vi "DIALOG_Cluster Item Selection.vi"(7 "Action":T4=enum."Bundler Insert", 8 "Error In":errorcluster, 9 "User VI Ref":refnum<vi>, 10 "Affected Items":T2, 11 "Display Items":T3[](array[typedef])) -> (0 "Error Out":errorcluster, 1 "Hide Full Names Out":bool=TRUE, 2 "Action Choice Out":enum32{"Choice 1", "Choice 2"}(radio), 3 "Selected Items (tags)":string[](array[string]))   [LabVIEW 2023]
doc: "Dialog to select items from the input cluster ref. \n\nFilter narrows list of items.\nDown key puts focus on tree and selects first item.\nUp and Down keps navigate tree.\nMultiple items can be selected.\n\nIn case of action \"Delete\" (\"Remove elements(s)...\" selected), list will show all elements currently displayed, else it will show all elements availabel to undle or unbundle.\n\nOutput is a list of the selected item tags.\n\nSelected element is the item clicked in a bundler node, displayed ot help user remember where an insert will happen."
uses:
  controls/Done Button.ctl
  controls/action enum.ctl
  cluster/Cluster Element Description.ctl
  top/BundleMagic.ctl
  utils/Controls/Get-Set Enum.ctl
  LabVIEW-common/String/Select All/String Select All CTRL-A_all string.vi
  <userlib>/_OpenG.lib/appcontrol/appcontrol.llb/openg_application_control.lvlib
  <userlib>/_OpenG.lib/error/error.llb/openg_error.lvlib
panel:
  in  "Filter":string
  in  "Tree":string[](tree)
  in  "Hide Full Names":bool=TRUE
  in  "Select Unwired":bool
  out "Selected Element String":string
  in  "Action Choice Radio Buttons":enum32{"Choice 1", "Choice 2"}(radio)
  in  "Done":T1
  in  "Show radio":bool
  in  "C1":T5
  # "All panes scroll to origin at runtime, so we don't have to worry about pane placements\n\nThis pane contracts at runtime and vertical splitter to left sticks to right at runtime so resizing functions happen as expected."
  # "Debug"
  # "Debug Cluster"
  # "(Use for debug if display items empty)"
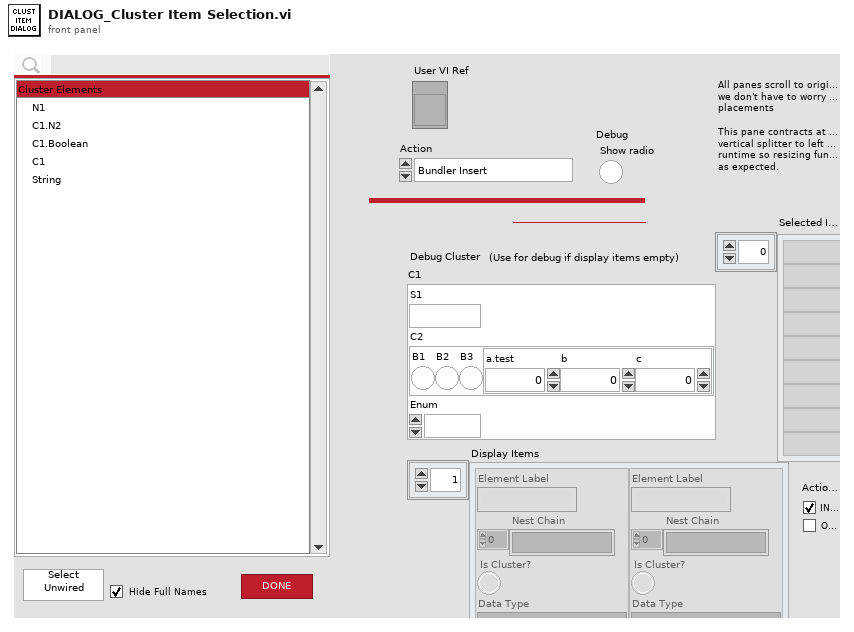
[diagram p1: front panel]
types:
  T1 = typedef "Done Button.ctl" = bool
  T2 = typedef "BundleMagic.ctl" = cluster{"Terminals":refnum<vi>[], "Wires":refnum<vi>[], "Named Bundler":refnum<vi>[], "Named Unbundler":refnum<vi>[], "In Place Cluster Node":refnum<vi>[], "Class Specifier Constant":refnum<vi>[], "Property Node":refnum<vi>[], "Invoke Node":refnum<vi>[], "Refnum Control":refnum<vi>[]}
  T3 = typedef "Cluster Element Description.ctl" = cluster{"Element Label":string, "Nest Chain":string[], "Is Cluster?":bool, "Data Type":variant, "Bundler Label":string, "Disabled":bool, "Unwired":bool, "Tree Tag":string}
  T4 = typedef "action enum.ctl" = enum16{"[NONE]", "APP_SEPARATOR", "Wire Bundle", "Wire Unbundle", "Terminal Unbundle", "Terminal Bundle", "Bundler Move Up", "Bundler Move Down", "Bundler Insert", "Bundler Remove", "Bundler Remove Unwired", "Bundler Reorder", "In Place Insert", "In Place Remove", "In Place Remove Unwired", "In Place Reorder", "Wire Properties", "Wire Method", "Terminal Properties", "Terminal Method", "Property Move Up", "Property Move Down", "Properties Insert", "Properties Remove", "Properties Remove Unwired", "Properties Reorder", "Method Change", "Class For Constant", "Class For Control", "Class For Node", "Class Name to Clipboard"}
  T5 = cluster{"S1":string, "C2":cluster{"B1":bool, "B2":bool, "B3":bool, cluster{"a.test":dbl, "b":i32, "c":u8}}, "Enum":enum16{""}}
  T6 = typedef "Get-Set Enum.ctl" = enum16{"Get", "Set"}
  T7 = typedef "LVPoint32TypeDef.ctl" = cluster{"Horizontal":i32, "Vertical":i32}
  T8 = cluster{"Shift":bool, "Ctrl":bool, "Alt":bool, "Cmd":bool, "Opt":bool}
  T9 = typedef "eventvkey.ctl" = enum16{"ASCII", "Enter", "Return", "Shift", "Ctrl", "Alt", "Cmd", "Opt", "Caps", "NumLock", "Clear", "Break", "Up", "Down", "Left", "Right", "Insert", "Delete", "Home", "End", "PageUp", "PageDown", "Escape", "Help", "Pause", "ScrollLock", "F1", "F2", "F3", "F4", "F5", "F6", "F7", "F8", "F9", "F10", "F11", "F12", "F13", "F14", "F15", "F16", "F17", "F18", "F19", "F20", "F21", "F22", "F23", "F24", "Play", "VolumeUp", "VolumeDown", "Mute", "Two Byte Char"}
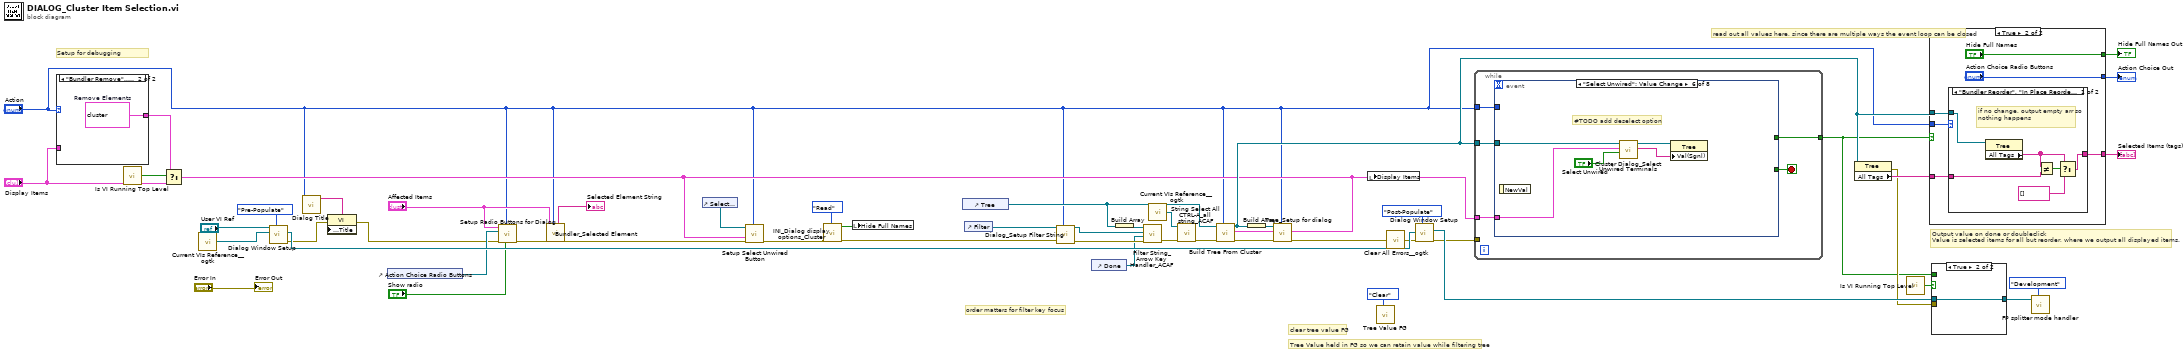
[diagram p0: block diagram]
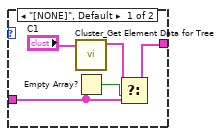
[diagram p2: hidden frame]
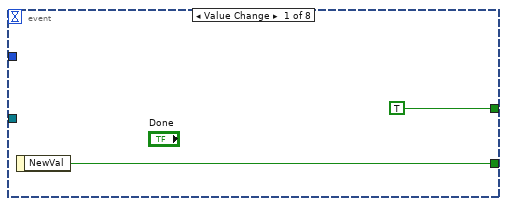
[diagram p3: hidden frame]
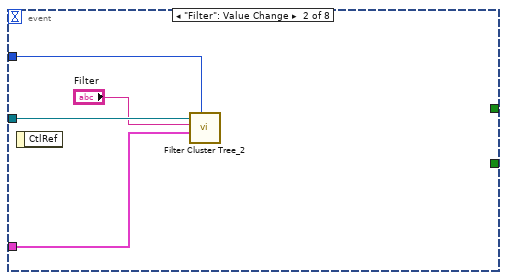
[diagram p4: hidden frame]
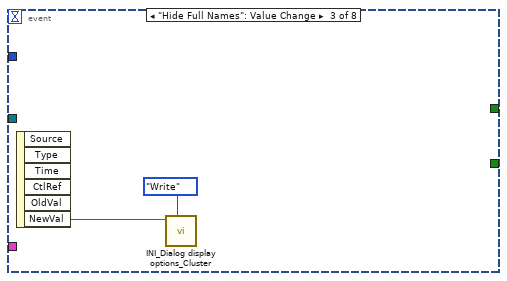
[diagram p5: hidden frame]
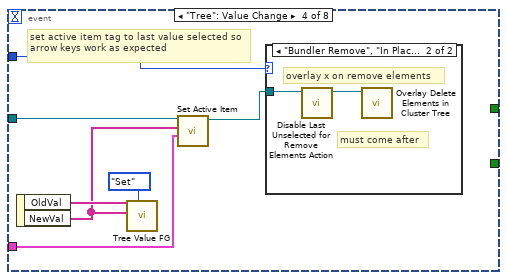
[diagram p6: hidden frame]
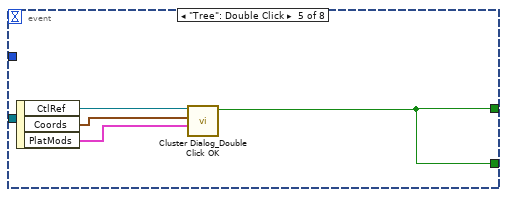
[diagram p8: hidden frame]
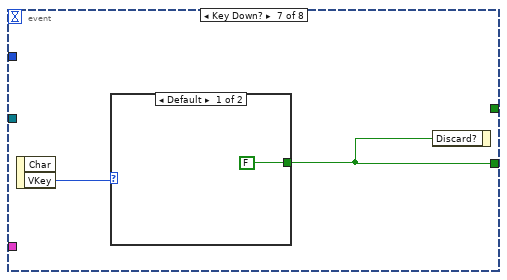
[diagram p9: hidden frame]
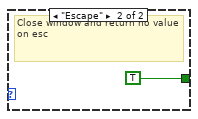
[diagram p10: hidden frame]
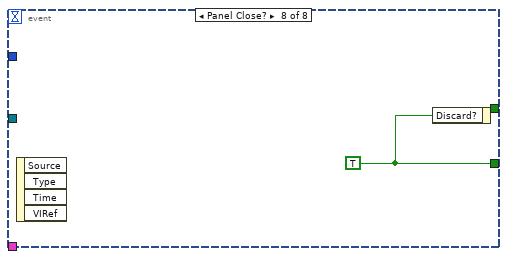
[diagram p11: hidden frame]
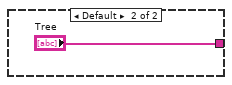
[diagram p13: hidden frame]
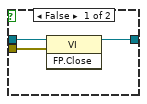
[diagram p14: hidden frame]
diagram:
  # "order matters for filter key focus"
  # "clear tree value FG"
  # "Setup for debugging"
  # "Tree Value held in FG so we can retain value while filtering tree"
  # "read out all values here, since there are multiple ways the event loop can be closed"
  # "Output value on done or doubleclick\nValue is selected items for all but reorder, where we output all displayed items."
  n1 = case shown="\"Bundler Remove\"..\"Bundler Reorder\"" "Action" {
    tunnel: [w55 w57] -> w40
    tunnel: "Display Items" -> [w54 _]
    frame "[NONE]", Default {
      n2 = call "Cluster_Get Element Data for Tree.vi"("Data Type"="C1") -> ("Cluster Element Data Aray"=w56:T3[])  [unwired: 10 in]
      n3 = Empty Array?(array=w54) -> (empty?=w53:bool)
      n4 = Select(t=w56, s=w53, f=w54) -> (s? t:f=w55:T3[])
    }
    frame "Bundler Remove".."Bundler Reorder" {
      w57 = T3[] [{"Element Label"="N1", "Nest Chain"=[], "Is Cluster?"=FALSE, "Data Type"=variant(dbl 0.0), "Bundler Label"="N1", "Disabled"=FALSE, "Unwired"=FALSE, "Tree Tag"="0[$`~g;}N1"}, {"Element Label"="N2", "Nest Chain"=["C1"], "Is Cluster?"=TRUE, "Data Type"=variant(dbl 0.0), "Bundler Label"="C1.N2", "Disabled"=FALSE, "Unwired"=FALSE, "Tree Tag"="C1[$`~g;}C1[$`~g;}N2"}, {"Element Label"="Boolean", "Nest Chain"=["C1"], "Is Cluster?"=TRUE, "Data Type"=variant(bool FALSE), "Bundler Label"="C1.Boolean", "Disabled"=FALSE, "Unwired"=TRUE, "Tree Tag"="C2[$`~g;}C1[$`~g;}Boolean"}, {"Element Label"="C1", "Nest Chain"=[], "Is Cluster?"=FALSE, "Data Type"=variant(cluster{"N2":dbl, "Boolean":bool} {"N2"=0.0, "Boolean"=FALSE}), "Bundler Label"="C1", "Disabled"=FALSE, "Unwired"=FALSE, "Tree Tag"="3[$`~g;}C1"}, {"Element Label"="String", "Nest Chain"=[], "Is Cluster?"=FALSE, "Data Type"=variant(string ""), "Bundler Label"="String", "Disabled"=FALSE, "Unwired"=FALSE, "Tree Tag"="4[$`~g;}String"}]  # Remove Elements
    }
  }
  n5 = call "Is VI Running Top Level.vi"() -> ("Top Level?"=w41:bool)  [unwired: 5 in]
  n6 = Select(t=w40, s=w41, f="Display Items") -> (s? t:f=w13:T3[])
  n7 = call <userlib>:"Current VIs Reference__ogtk.vi"() -> ("Current VI's reference"=w20:refnum<vi>)  [unwired: 5 in]
  n8 = call "Dialog Window Setup.vi"("Action"=enum16{"Pre-Populate", "Post-Populate"}."Pre-Populate", "Dialog VI Ref In [Parent]"=w20, "Align-to Window Ref"="User VI Ref") -> ("error out"=w18:errorcluster, "Dialog VI Ref Out"=w45:refnum<vi>)  [unwired: 7 in]
  n9 = call "Dialog Title.vi"("Action"="Action") -> ("Window Title"=w26:string)  [unwired: 10 in]
  n10 = property class="VI"(error in=w18, "Front Panel.Title"=w26) -> (error out=w17:errorcluster)  [unwired: 1 in, 1 out]
  n11 = control-ref of="Action Choice Radio Buttons"() -> (w28:refnum<vi>)
  n12 = call "Setup Radio Buttons for Dialog.vi"("Show Radio"="Show radio", "Action"="Action", "error in (no error)"=w17, "Action Choice Ref"=w28, "Affected Items"="Affected Items") -> ("error out"=w16:errorcluster)  [unwired: 6 in]
  n13 = call "Bundler_Selected Element.vi"("Action"="Action", "error in (no error)"=w16, "Affected Items"="Affected Items") -> ("error out"=w15:errorcluster, "Display String"=→"Selected Element String":string)  [unwired: 2 in, 5 out]
  n14 = control-ref of="Select Unwired"() -> (w27:refnum<vi>)
  n15 = call "Setup Select Unwired Button.vi"("Action"="Action", "error in (no error)"=w15, "Display Items"=w13, "Boolean in"=w27) -> ("error out"=w4:errorcluster)  [unwired: 7 in]
  n16 = call "INI_Dialog display options_Cluster.vi"("File Action"=enum16{"Read", "Write"}."Read", "error in (no error)"=w4) -> ("error out"=w3:errorcluster, "Hide Full Names Out"=w2:bool)  [unwired: 8 in]
  n17 = local write "Hide Full Names"(w2) -> ()
  n18 = control-ref of="Tree"() -> (w12:refnum<vi>)
  n19 = control-ref of="Filter"() -> (w21:refnum<vi>)
  n20 = call "Dialog_Setup Filter String.vi"("Action"="Action", "error in"=w3, "Filter String Ref"=w21) -> ("error out"=w11:errorcluster, "Filter String Ref Out"=w7:refnum<vi>)  [unwired: 7 in]
  n21 = control-ref of="Done"() -> (w9:refnum<vi>)
  n22 = Build Array(w12) -> (w8:refnum<vi>[])
  n23 = call "Filter String_Arrow Key Handler_ACAF.vi"("error in (no error)"=w11, "Done Ref"=w9, "Filter String Ref"=w7, "Tree Ref Array"=w8) -> ("error out"=w10:errorcluster)  [unwired: 7 in]
  n24 = call <userlib>:"Current VIs Reference__ogtk.vi"() -> ("Current VI's reference"=w19:refnum<vi>)  [unwired: 5 in]
  n25 = call "String Select All CTRL-A_all string_ACAF.vi"("error in (no error)"=w10, "VI Ref"=w19) -> ("error out"=w36:errorcluster)  [unwired: 9 in]
  n26 = call "Build Tree From Cluster.vi"("Action"="Action", "error in"=w36, "Display Items"=w13, "Tree Ref"=w12) -> ("error out"=w35:errorcluster, "Tree Ref Out"=w42:refnum<vi>)  [unwired: 6 in]
  n27 = Build Array(w42) -> (w34:refnum<vi>[])
  n28 = call "Tree_Setup for dialog.vi"("Action"="Action", "error in"=w35, "Tree Ref"=w34) -> ("error out"=w33:errorcluster)  [unwired: 7 in, 1 out]
  n29 = local write "Display Items"(w13) -> ()
  n30 = call "Tree Value FG.vi"("Get Set Enum"=enum16{"Get", "Set", "Clear"}."Clear") -> ()  [unwired: 10 in, 1 out]
  n31 = call <userlib>:"Clear All Errors__ogtk.vi"("Error In"=w33) -> ("Error Out"=w31:errorcluster)  [unwired: 3 in]
  n32 = call "Dialog Window Setup.vi"("Action"=enum16{"Pre-Populate", "Post-Populate"}."Post-Populate", "error in"=w31, "Dialog VI Ref In [Parent]"=w45) -> ("error out"=w43:errorcluster, "Dialog VI Ref Out"=w44:refnum<vi>)  [unwired: 7 in]
  n33 = while {
    tunnel: w42 -> [w61]
    tunnel: [w60] -> w37
    tunnel: "Action" -> [w59]
    tunnel: w13 -> [w58]
    tunnel: w43 -> [_]
    stop <- w62 stop-if-true
    n34 = event shown="[5] \"Select Unwired\": Value Change" {
      selector: _ -> [_ _ _ _ _ _ _ _]
      dyn-events: _ -> [_ _ _ _ _ _ _ _]
      timeout: _ -> [_ _ _ _ _ _ _ _]
      tunnel: [w64 _ _ _ w83 _ w89 w93] -> w62
      tunnel: w61 -> [_ w68 _ w75 _ w87 _ _]
      tunnel: [TRUE _ _ _ w83 _ _ _] -> w60
      tunnel: w59 -> [_ w65 _ w77 _ _ _ _]
      tunnel: w58 -> [_ w66 _ w71 _ w88 _ _]
      event Value Change {
        n35 = event-data() -> ("NewVal"=w64:T1)  [unwired: 1 in]
      }
      event "Filter": Value Change {
        n36 = event-data() -> ()  [unwired: 1 in, 1 out]
        n37 = call "Filter Cluster Tree_2.vi"("Action"=w65, "Display Items"=w66, "Filter Str"="Filter", "Tree Ref"=w68) -> ()  [unwired: 7 in, 1 out]
      }
      event "Hide Full Names": Value Change {
        n38 = event-data() -> ("NewVal"=w69:bool)  [unwired: 1 in, 5 out]
        n39 = call "INI_Dialog display options_Cluster.vi"("File Action"=enum16{"Read", "Write"}."Write", "Hide Full Names"=w69) -> ()  [unwired: 8 in, 2 out]
      }
      event "Tree": Value Change {
        # "set active item tag to last value selected so arrow keys work as expected"
        n40 = event-data() -> ("OldVal"=w74:string[], "NewVal"=w72:string[])  [unwired: 1 in]
        n41 = call "Tree Value FG.vi"("Get Set Enum"=Get-Set_Enum."Set", "NewVal"=w72, "Old Val"=w74) -> ()  [unwired: 8 in, 1 out]
        n42 = call "Set Active Item.vi"("Display Items"=w71, "NewVal"=w72, "TreeControl in"=w75) -> ("TreeControl out"=w76:refnum<vi>)  [unwired: 8 in]
        n43 = case shown="\"Bundler Remove\", \"In Place Remove\"" w77 {
          tunnel: w76 -> [_ w79]
          frame "[NONE]", Default {
          }
          frame "Bundler Remove", "In Place Remove" {
            # "overlay x on remove elements"
            # "must come after"
            n44 = call "Disable Last Unselected for Remove Elements Action.vi"("Tree Ref"=w79) -> ("Tree Ref Out"=w78:refnum<vi>)  [unwired: 8 in, 2 out]
            n45 = call "Overlay Delete Elements in Cluster Tree.vi"("Tree Ref"=w78) -> ()  [unwired: 10 in, 1 out]
          }
        }
      }
      event "Tree": Double Click {
        # "Double click to select and end entry"
        n46 = event-data() -> ("CtlRef"=w82:refnum<vi>, "Coords"=w81:T7, "PlatMods"=w80:T8)  [unwired: 1 in]
        n47 = call "Cluster Dialog_Double Click OK.vi"("PlatMods"=w80, "Coords"=w81, "TreeControl in"=w82) -> ("Valid Item Double Clicked"=w83:bool)  [unwired: 8 in]
      }
      event "Select Unwired": Value Change {
        # "#TODO add deselect option"
        n48 = event-data() -> ()  [unwired: 1 in, 1 out]
        n49 = call "Cluster Dialog_Select Unwired Terminals.vi"("Select Unwired"="Select Unwired", "Display Items"=w88, "Tree Ref"=w87) -> ("Selected items"=w84:string[], "Tree Ref Out"=w85:refnum<vi>)  [unwired: 7 in]
        n50 = property class="Tree"(reference=w85, "Val(Sgnl)"=w84) -> ()  [unwired: 1 in, 2 out]
      }
      event Key Down? {
        # "Quit on escape"
        n51 = event-data() -> ("VKey"=w90:T9)  [unwired: 1 in, 1 out]
        n52 = case shown="Default" w90 {
          tunnel: [FALSE TRUE] -> w89
          frame Default {
          }
          frame "Escape" {
            # "Close window and return no value on esc"
          }
        }
        n53 = event-data("Discard?"=w89) -> ()  [unwired: 1 in, 1 out]
      }
      event Panel Close? {
        w93 = TRUE
        # "close and return no value on panel close"
        n54 = event-data() -> ()  [unwired: 1 in, 4 out]
        n55 = event-data("Discard?"=w93) -> ()  [unwired: 1 in, 1 out]
      }
    }
  }
  n56 = property class="Tree"(reference=w42) -> (error out=w38:errorcluster, "All Tags"=w46:string[])  [unwired: 1 in, 1 out]
  n57 = call "Is VI Running Top Level.vi"() -> ("Top Level?"=w48:bool)  [unwired: 5 in]
  n58 = case shown="True" w37 {
    tunnel: [_ w99] -> w51
    tunnel: "Action" -> [_ w98]
    tunnel: w42 -> [_ w97]
    tunnel: [_ "Action Choice Radio Buttons"] -> w49
    tunnel: w46 -> [_ w95]
    tunnel: [_ "Hide Full Names"] -> w1
    frame False {
    }
    frame True {
      n59 = case shown="\"Bundler Reorder\", \"In Place Reorder\"" w98 {
        tunnel: [w100 "Tree"] -> w99
        tunnel: w97 -> [w105 _]
        tunnel: w95 -> [w104 _]
        frame "Bundler Reorder", "In Place Reorder" {
          # "if no change, output empty arr so nothing happens"
          n60 = property class="Tree"(reference=w105) -> ("All Tags"=w101:string[])  [unwired: 1 in, 2 out]
          n61 = Not Equal?(x=w101, y=w104) -> (x != y?=w103:bool)
          n62 = Select(t=w101, s=w103, f=string[] []) -> (s? t:f=w100:string[])
        }
        frame Default {
        }
      }
    }
  }
  "Selected Items (tags)" <- w51
  "Action Choice Out" <- w49
  "Hide Full Names Out" <- w1
  n63 = case shown="True" w48 {
    tunnel: w44 -> [w109 w110]
    tunnel: [w108 w110] -> w47
    tunnel: w38 -> [w107 _]
    tunnel: w37 -> [_ _]
    frame False {
      n64 = invoke class="VI" method="FP.Close"(reference=w109, error in=w107) -> (reference out=w108:refnum<vi>)  [unwired: 1 in, 2 out]
    }
    frame True {
    }
  }
  n65 = call "FP splitter mode handler.vi"("Mode"=enum16{"Run", "Development"}."Development", "VI Ref In"=w47) -> ()  [unwired: 8 in, 2 out]
  "Error Out" <- "Error In"
